vi "sReg Min Max.vi"(2 "Max from sReg":i32, 3 "New Value":i32, 4 "Min from sReg":i32) -> (0 "Max to sReg":i32, 1 "Min to sReg":i32)   [LabVIEW 2010]
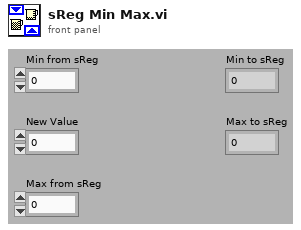
[diagram p1: front panel]
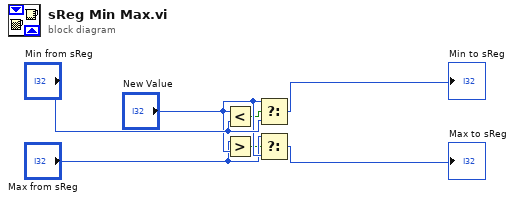
[diagram p0: block diagram]
diagram:
  n1 = Less?(x="New Value", y="Min from sReg") -> (x < y?=w4:bool)
  n2 = Greater?(x="Max from sReg", y="New Value") -> (0:w1:bool)
  n3 = Select(t="New Value", s=w4, f="Min from sReg") -> (s? t:f=→"Min to sReg":i32)
  n4 = Select(t="Max from sReg", s=w1, f="New Value") -> (s? t:f=→"Max to sReg":i32)
